vi "SMBus Hard Init.vi"(6 "OwnAddr":u8, 7 "ClockSpeed":u32, 9 "SMBUSIndex":i32, 10 "DevIndex":i32, 11 "DevType":i32) -> (3 "function return":i32)   [LabVIEW 2010, in "ControlSMBus.lvlib"]
doc: "int WINAPI SMBus_HardInit(int DevType,int DevIndex,int SMBUSIndex,unsigned int ClockSpeed, unsigned char OwnAddr);"
uses:
  ControlSMBus.lvlib
  ControlSMBus/Ginkgo_Driver.dll
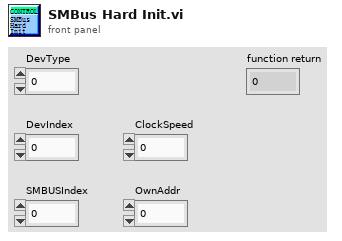
[diagram p1: front panel]
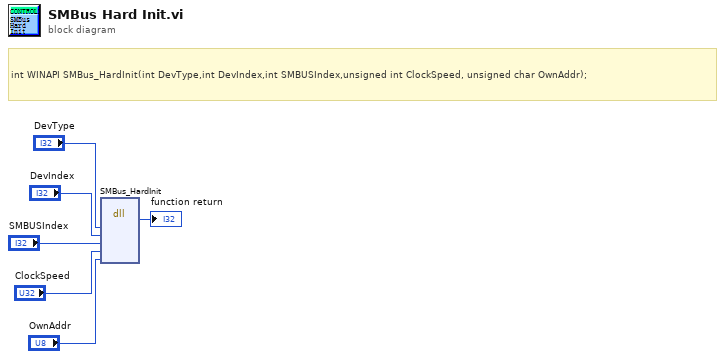
[diagram p0: block diagram]
diagram:
  # "int WINAPI SMBus_HardInit(int DevType,int DevIndex,int SMBUSIndex,unsigned int ClockSpeed, unsigned char OwnAddr);"
  n1 = dll-call lib="E:/Project/vt_ginkgo/truck/Ginkgo Driver/vs2010/Ginkgo_USB-I2C&SPI&CAN_API_v2.0.3.3/lib/labview_32bit/ControlSMBus/Ginkgo_Driver.*" fn="SMBus_HardInit"("DevType"="DevType", "DevIndex"="DevIndex", "SMBUSIndex"="SMBUSIndex", "ClockSpeed"="ClockSpeed", "OwnAddr"="OwnAddr") -> (→"function return":i32)  [unwired: 8 in, 2 out]
